vi "Create AUTH Packet.vi"(5 "AUTH in":refnum<class "AUTH.lvclass">, 8 "error in (no error)":errorcluster) -> (0 "error out":errorcluster, 3 "AUTH":refnum<class "AUTH.lvclass">)   [LabVIEW 2013, in "MQTT_Control_Packets_50.lvlib" / "AUTH.lvclass"]
uses:
  AUTH.lvclass
  ControlPacket/ControlPacket.lvclass/ControlPacket.ctl
  ControlPacket/ControlPacket.lvclass
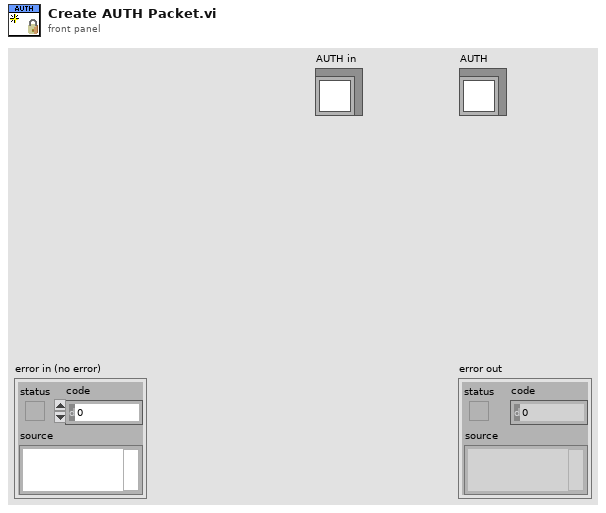
[diagram p1: front panel]
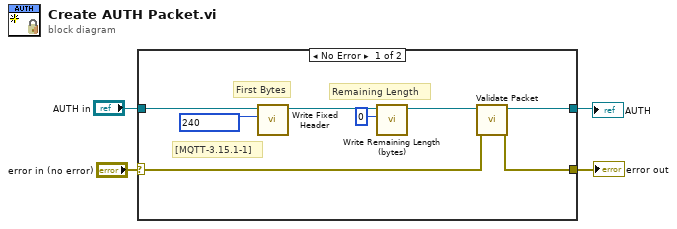
[diagram p0: block diagram]
diagram:
  n1 = case shown="No Error" "error in (no error)" {
    selector: "error in (no error)" -> [w6 w14]
    tunnel: [w5 w14] -> w1
    tunnel: [w7 w13] -> w2
    tunnel: "AUTH in" -> [w12 w13]
    frame No Error {
      # "[MQTT-3.15.1-1]"
      # "Remaining Length"
      # "First Bytes"
      n2 = call "Write Fixed Header.vi"("Fixed Header"=u8 240, "ControlPacket in"=w12) -> ("ControlPacket out"=w11:refnum<class "AUTH.lvclass">)  [unwired: 9 in]
      n3 = call "Write Remaining Length (bytes).vi"("Remaining Length (bytes)"=u32 0, "ControlPacket in"=w11) -> ("ControlPacket out"=w8:refnum<class "AUTH.lvclass">)  [unwired: 9 in]
      n4 = call "Validate Packet.vi"("error in (no error)"=w6, "ControlPacket in"=w8) -> ("error out"=w5:errorcluster, "ControlPacket out"=w7:refnum<class "AUTH.lvclass">)  [unwired: 8 in]
    }
    frame Error {
    }
  }
  "error out" <- w1
  "AUTH" <- w2
